vi "Compile Event Capture 1.0 Data.vi"(7 "RIO Address":string, 8 "error in (no error)":errorcluster, 11 "Device Item Ref in":T3 format="%.0x") -> (0 "error out":errorcluster, 2 "Event Timing Captures":T1[](array[typedef]), 3 "Device Item Ref out":T3 format="%.0x")   [LabVIEW 2020, in "Engine Simulation Toolkit System Explorer.lvlib"]
uses:
  Engine Simulation Toolkit System Explorer.lvlib
  <vilib>/NI VeriStand/Custom Device API/Custom Device Item Ref.ctl
  Shared/1.0 Event Timing Capture Engine Data.ctl
  Shared/1.0 Event Timing Capture FIFO Idxs.ctl
  Shared/Constants and GUIDs.vi
  <vilib>/NI VeriStand/Custom Device Tools/Custom Device Utility Library/NI VeriStand - Search for Item by GUID.vi
  Shared/Properties.vi
  <vilib>/NI VeriStand/Custom Device API/Get Item Property (String).vi
  Shared/Engine Simulation Toolkit Shared.lvlib
  <vilib>/NI VeriStand/Custom Device Tools/Custom Device Utility Library/Custom Device Utility Library.lvlib
  <vilib>/NI VeriStand/Custom Device API/Custom Device API.lvlib
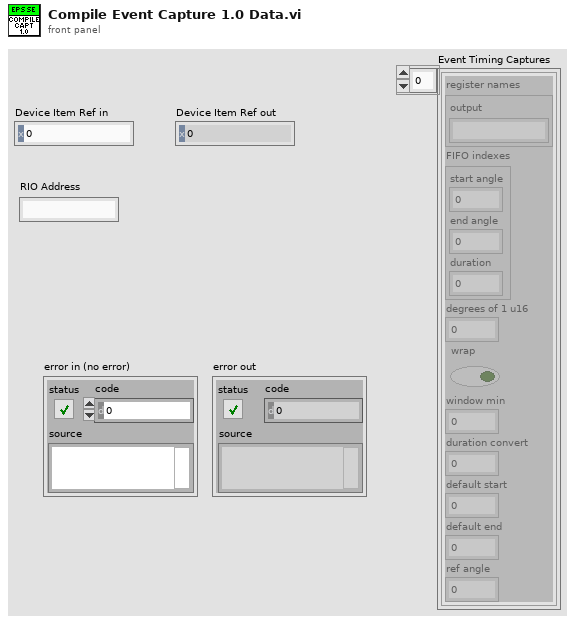
[diagram p1: front panel]
types:
  T1 = typedef "Engine Simulation Toolkit Shared.lvlib/1.0 Event Timing Capture Engine Data.ctl" = cluster{"register names":cluster{"output":string}, "FIFO indexes":T2, "degrees of 1 u16":dbl, "wrap":bool, "window min":u16, "duration convert":dbl, "default start":dbl, "default end":dbl, "ref angle":dbl}
  T2 = typedef "Engine Simulation Toolkit Shared.lvlib/1.0 Event Timing Capture FIFO Idxs.ctl" = cluster{"start angle":i32, "end angle":i32, "duration":i32}
  T3 = typedef "Custom Device API.lvlib/Custom Device Item Ref.ctl" = u64
  T4 = typedef "Engine Simulation Toolkit Shared.lvlib/Channel.ctl" = cluster{"Name":string, "Units":string, "Default":dbl, "Description":string, "Scalable":bool}
  T5 = typedef "Engine Simulation Toolkit System Explorer.lvlib/Event Timing Window.ctl" = cluster{"Name":string, "Min":dbl, "Max":dbl, "Ref":dbl}
  T6 = typedef "Engine Simulation Toolkit System Explorer.lvlib/Event Timing Capture.ctl" = cluster{"Name":string, "Bitfile name":string, "Reference angle":dbl, "Default start":dbl, "Default end":dbl, "Ref Select":T7}
  T7 = typedef "Engine Simulation Toolkit System Explorer.lvlib/Event Reference Angle Selection.ctl" = enum16{"From window", "Custom"}
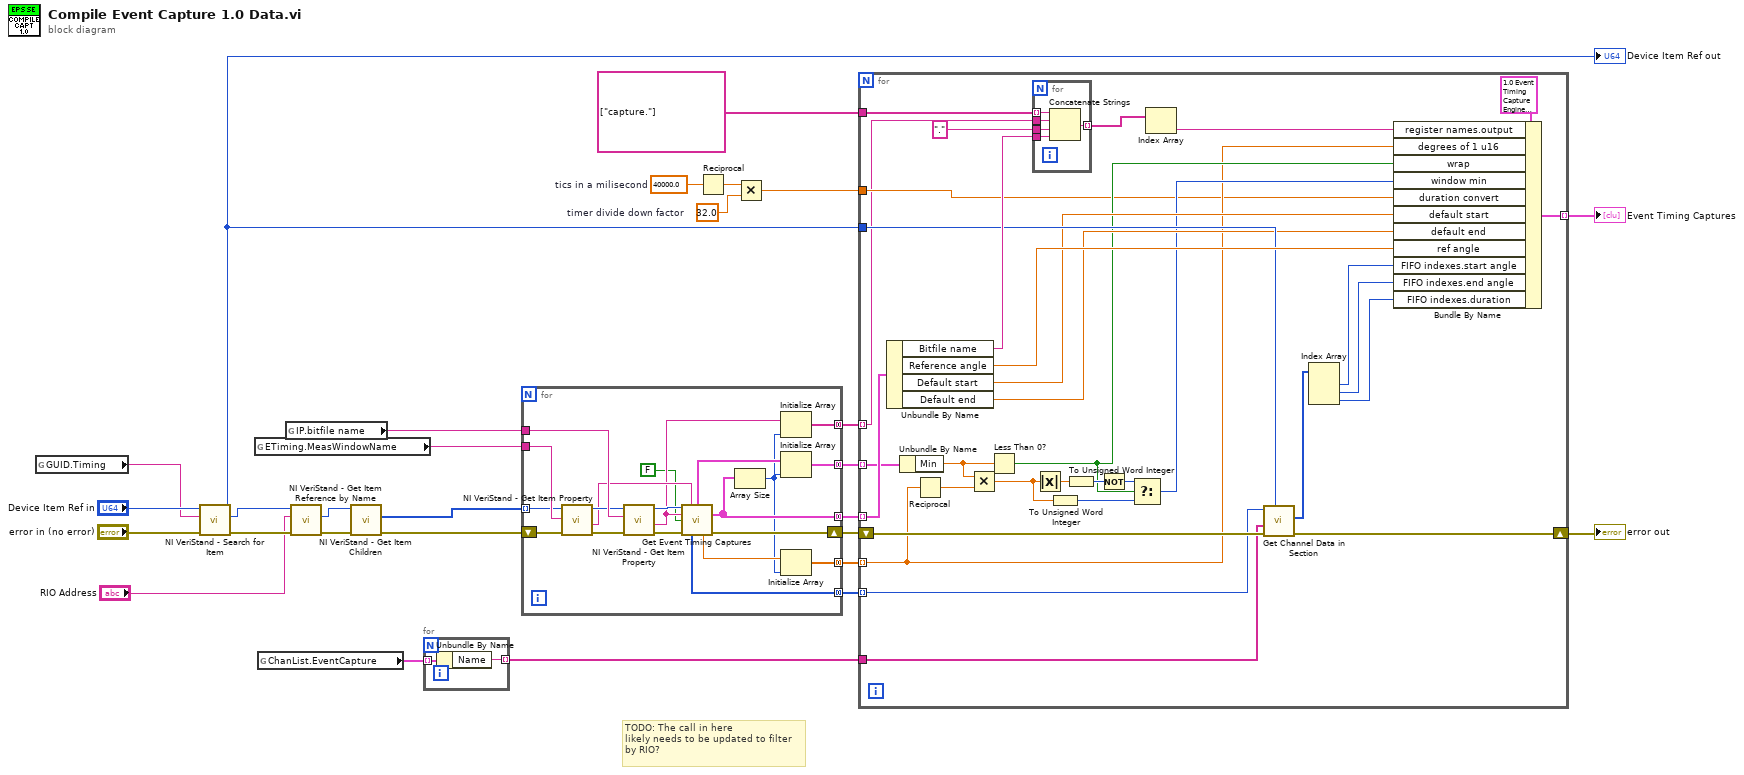
[diagram p0: block diagram]
diagram:
  w9 = 32.0  # timer divide down factor
  w11 = 40000.0  # tics in a milisecond
  # "TODO: The call in here\nlikely needs to be updated to filter\nby RIO?"
  n1 = global read "Constants and GUIDs.vi" "GUID.Timing"() -> (w19:string)
  n2 = call-poly <vilib>:"NI VeriStand - Search for Item.vi"("error in"="error in (no error)", "Item GUID"=w19, "Section Ref in"="Device Item Ref in") -> ("error out"=w25:errorcluster, "Item Ref"=w4:T3, "Section Ref out"=w2:T3)  [unwired: 5 in, 1 out]
  "Device Item Ref out" <- w2
  n3 = global read "Properties.vi" "ETiming.MeasWindowName"() -> (w17:string)
  n4 = global read "Constants and GUIDs.vi" "ChanList.EventCapture"() -> (w21:T4[])
  n5 = global read "Properties.vi" "IP.bitfile name"() -> (w16:string)
  n6 = call <vilib>:"NI VeriStand - Get Item Reference by Name.vi"("Item Name"="RIO Address", "Parent Ref in"=w4) -> ("error out"=w5:errorcluster, "Item Ref"=w6:T3)  [unwired: 6 in, 2 out]
  n7 = call <vilib>:"NI VeriStand - Get Item Children.vi"("error in (no error)"=w5, "Item Ref in"=w6) -> ("Child Refs"=w1:T3[])  [unwired: 6 in, 3 out]
  n8 = for {
    tunnel: w21 -> [w29] mode=indexing
    tunnel: [w28] -> w20 mode=indexing
    n9 = Unbundle By Name(w29) -> ("Name"=w28:string)
  }
  n10 = for {
    tunnel: w1 -> [w33] mode=indexing
    shift-right: [w44] -> w18
    shift-left: w25 -> [w49]
    tunnel: w17 -> [w46]
    tunnel: w16 -> [w45]
    tunnel: [w38] -> w15 mode=concatenating
    tunnel: [w41] -> w14 mode=concatenating
    tunnel: [w40] -> w13 mode=concatenating
    tunnel: [w37] -> w12 mode=concatenating
    tunnel: [w35] -> w7 mode=concatenating
    n11 = call-poly <vilib>:"NI VeriStand - Get Item Property.vi"("error in (no error)"=w49, "Property Name"=w46, "Item Ref in"=w33) -> ("error out"=w48:errorcluster, "Value"=w32:string, "Item Ref out"=w34:T3)  [unwired: 5 in, 1 out]
    n12 = call-poly <vilib>:"NI VeriStand - Get Item Property.vi"("error in (no error)"=w48, "Property Name"=w45, "Item Ref in"=w34) -> ("error out"=w47:errorcluster, "Value"=w31:string, "Item Ref out"=w43:T3)  [unwired: 5 in, 1 out]
    n13 = call "Get Event Timing Captures.vi"("Item Ref in"=w43, "Window"=w32, "Timing measurement"=w31, "return all captures (T)"=FALSE, "error in (no error)"=w47) -> ("window"=w39:T5, "captures"=w38:T6[], "Capture item refs"=w40:T3[], "degrees of one u16"=w42:dbl, "error out"=w44:errorcluster)  [unwired: 2 in, 4 out]
    n14 = Array Size(array=w38) -> (size(s)=w36:i32)
    n15 = Initialize Array(w31, w36) -> (w35:string[])
    n16 = Initialize Array(w39, w36) -> (w37:T5[])
    n17 = Initialize Array(w42, w36) -> (w41:dbl[])
  }
  n18 = Reciprocal(x=w11) -> (1/x=w10:dbl)
  n19 = Multiply(x=w10, y=w9) -> (x*y=w8:dbl)
  n20 = for {
    shift-right: [w70] -> w23
    shift-left: w18 -> [w74]
    tunnel: string[] ["capture."] -> [w82]
    tunnel: w20 -> [w71]
    tunnel: [w80] -> w22 mode=indexing
    tunnel: w2 -> [w72]
    tunnel: w15 -> [w79] mode=indexing
    tunnel: w14 -> [w54] mode=indexing
    tunnel: w13 -> [w73] mode=indexing
    tunnel: w12 -> [w63] mode=indexing
    tunnel: w8 -> [w52]
    tunnel: w7 -> [w50] mode=indexing
    n21 = Unbundle By Name(w79) -> ("Bitfile name"=w78:string, "Reference angle"=w75:dbl, "Default start"=w65:dbl, "Default end"=w64:dbl)
    n22 = Unbundle By Name(w63) -> ("Min"=w56:dbl)
    n23 = Reciprocal(x=w54) -> (1/x=w53:dbl)
    n24 = Multiply(x=w56, y=w53) -> (x*y=w55:dbl)
    n25 = Less Than 0?(x=w56) -> (x < 0?=w58:bool)
    n26 = for {
      tunnel: w82 -> [w87] mode=indexing
      tunnel: [w83] -> w77 mode=indexing
      tunnel: w78 -> [w86]
      tunnel: w50 -> [w85]
      tunnel: "." -> [w84]
      n27 = Concatenate Strings(w87, w85, w84, w86) -> (w83:string)
    }
    n28 = Absolute Value(x=w55) -> (abs(x)=w60:dbl)
    n29 = To Unsigned Word Integer(number=w55) -> (unsigned 16bit integer=w62:u16)
    n30 = To Unsigned Word Integer(number=w60) -> (unsigned 16bit integer=w59:u16)
    n31 = Not(x=w59) -> (.not. x?=w61:u16)
    n32 = Select(t=w61, s=w58, f=w62) -> (s? t:f=w57:u16)
    n33 = Index Array(array=w77) -> (element=w76:string)  [unwired: 1 in]
    n34 = call "Get Channel Data in Section.vi"("Custom device ref"=w72, "error in (no error)"=w74, "Channels"=w71, "Item Ref in"=w73) -> ("error out"=w70:errorcluster, "FIFO indexes"=w69:i32[])  [unwired: 3 in, 3 out]
    n35 = Index Array(array=w69) -> (element #1=w68:i32, element #2=w67:i32, element #3=w66:i32)  [unwired: 3 in]
    n36 = Bundle By Name(cluster=T1 {"register names"={"output"=""}, "FIFO indexes"={"start angle"=0, "end angle"=0, "duration"=0}, "degrees of 1 u16"=0.0, "wrap"=FALSE, "window min"=0, "duration convert"=0.0, "default start"=0.0, "default end"=0.0, "ref angle"=0.0} ("1.0.0 Event Timing Capture"), "register names.output"=w76, "degrees of 1 u16"=w54, "wrap"=w58, "window min"=w57, "duration convert"=w52, "default start"=w65, "default end"=w64, "ref angle"=w75, "FIFO indexes.start angle"=w68, "FIFO indexes.end angle"=w67, "FIFO indexes.duration"=w66) -> (w80:T1)
  }
  "error out" <- w23
  "Event Timing Captures" <- w22
